vi "ULtravolt_Test_V1.3.vi"() -> ()   [LabVIEW 2022 SP3]
panel:
  out "UltraVolt Pout":dynamicdata(graph)=[{"t0"=timestamp(3793121458.353568 s since 1904-01-01), "dt"=0.004, "Y"=[0.002604330009442325, 0.0025504771878336083, 0.002568428128369847, 0.002532775426754479, 0.00251507366567535, 0.0024973719045962212, 0.0024973719045962212, 0.002550601777562163, 0.002568428128369847, 0.002586254479177531, 0.002604330009442325, 0.00275042932830334, 0.002604080829985215, 0.002358000431077182, 0.0020747622341868144, 0.001841629147424206, 0.0018114583938652624, 0.0017221920304739823, 0.0017667006224410674, 0.001737152817524899, 0.001737152817524899, 0.0016930179947434792, 0.0017518644251187055, 0.0017224412099310924, 0.0017224412099310924, 0.0016643423179271966, 0.0017667006224410674, 0.0017221920304739823, 0.0017667006224410674, 0.0017667006224410674, 0.0017221920304739823, 0.001856839113932233, 0.0019803876919247754, 0.002223114187786126, 0.0024607224851524124, 0.0027501801488462293, 0.00275042932830334, 0.0026222809499785644, 0.002676632130501502, 0.0026402318905148032, 0.0025504771878336083, 0.0026222809499785644, 0.002550601777562163, 0.002568428128369847, 0.002604330009442325, 0.002604330009442325, 0.002604330009442325, 0.002604330009442325, 0.002604330009442325, 0.002568178948912737, 0.002514949075946795, 0.002462217561895074, 0.0024796701435170925, 0.0024973719045962212, 0.002532775426754479, 0.0026404810699719133, 0.0026950814299519614, 0.0026950814299519614, 0.0025858807099918657, 0.0023233444472902545, 0.0020437193525279854, 0.001826419180916179, 0.0017964976068143457, 0.0017667006224410674, 0.0017964976068143457, 0.0017518644251187055, 0.0017812876403063187, 0.0017224412099310924, 0.0017077296023372858, 0.0016932671742005893, 0.001737152817524899, 0.0017224412099310924, 0.0017077296023372858, 0.0016930179947434792, 0.0017518644251187055, 0.0017518644251187055, 0.0018114583938652624, 0.001841629147424206, 0.0019333873053865884, 0.002172999058034062, 0.002392407235406999, 0.002658556600236708, 0.0028061509958403836, 0.0026952060196805167, 0.002658182831051042, 0.002658556600236708, 0.002604330009442325, 0.0025858807099918657, 0.002604330009442325, 0.0025863790689060863, 0.002586254479177531, 0.002604330009442325, 0.002586254479177531, 0.0026222809499785644, 0.002568178948912737, 0.002568428128369847, 0.002568178948912737, 0.00251507366567535, 0.0024796701435170925, 0.002514949075946795], "attributes"=variant("NI_ChannelName"=variant(string "Eout (Ultravolt)"), "NI_UnitDescription"=variant(string "E-Volts"))}]
  out "UltraVolt Eout":dynamicdata(graph)=[{"t0"=timestamp(3793121458.353568 s since 1904-01-01), "dt"=0.004, "Y"=[-4.674759833142161, -4.642537981271744, -4.642537981271744, -4.578094277530909, -4.578094277530909, -4.545872425660491, -4.578094277530909, -4.610316129401326, -4.610316129401326, -4.610316129401326, -4.642537981271744, -4.771425388753414, -4.706981685012579, -4.481428721919656, -4.255875758826733, -3.9336572401225567, -3.901435388252139, -3.836991684511304, -3.836991684511304, -3.8047698326408863, -3.8047698326408863, -3.8047698326408863, -3.8047698326408863, -3.7725479807704687, -3.8047698326408863, -3.740326128900051, -3.836991684511304, -3.836991684511304, -3.836991684511304, -3.836991684511304, -3.740326128900051, -3.9336572401225567, -4.0303227957338095, -4.28809761069715, -4.416985018178821, -4.739203536882997, -4.803647240623832, -4.642537981271744, -4.771425388753414, -4.739203536882997, -4.642537981271744, -4.642537981271744, -4.610316129401326, -4.610316129401326, -4.642537981271744, -4.674759833142161, -4.674759833142161, -4.674759833142161, -4.674759833142161, -4.674759833142161, -4.545872425660491, -4.545872425660491, -4.513650573790073, -4.545872425660491, -4.578094277530909, -4.674759833142161, -4.706981685012579, -4.771425388753414, -4.706981685012579, -4.481428721919656, -4.15921020321548, -3.9336572401225567, -3.8692135363817215, -3.836991684511304, -3.8692135363817215, -3.8047698326408863, -3.8047698326408863, -3.8047698326408863, -3.8047698326408863, -3.7725479807704687, -3.8047698326408863, -3.8047698326408863, -3.740326128900051, -3.8047698326408863, -3.8047698326408863, -3.836991684511304, -3.901435388252139, -3.9336572401225567, -3.9658790919929743, -4.1914320550858974, -4.416985018178821, -4.674759833142161, -4.868090944364667, -4.739203536882997, -4.642537981271744, -4.739203536882997, -4.642537981271744, -4.578094277530909, -4.674759833142161, -4.642537981271744, -4.674759833142161, -4.674759833142161, -4.674759833142161, -4.642537981271744, -4.674759833142161, -4.642537981271744, -4.674759833142161, -4.578094277530909, -4.513650573790073, -4.545872425660491], "attributes"=variant("NI_ChannelName"=variant(string "Eout (Ultravolt)"), "NI_UnitDescription"=variant(string "E-Volts"))}]
  out "UltraVolt Iout":dynamicdata(graph)=[{"t0"=timestamp(3793121458.355568 s since 1904-01-01), "dt"=0.004, "Y"=[-0.5571045577526093, -0.549371313303709, -0.5532379355281591, -0.5532379355281591, -0.549371313303709, -0.549371313303709, -0.5455046910792589, -0.5532379355281591, -0.5571045577526093, -0.5609711799770594, -0.5609711799770594, -0.5764376688748598, -0.5532379355281591, -0.5261715799570084, -0.48750535771250725, -0.4681722465902567, -0.4643056243658066, -0.44883913546800613, -0.46043900214135647, -0.45657237991690636, -0.45657237991690636, -0.444972513243556, -0.46043900214135647, -0.45657237991690636, -0.45270575769245625, -0.444972513243556, -0.46043900214135647, -0.44883913546800613, -0.46043900214135647, -0.46043900214135647, -0.46043900214135647, -0.4720388688147068, -0.49137197993695736, -0.5184383355081081, -0.5571045577526093, -0.5803042910993099, -0.5725710466504097, -0.5648378022015095, -0.5609711799770594, -0.5571045577526093, -0.549371313303709, -0.5648378022015095, -0.5532379355281591, -0.5571045577526093, -0.5609711799770594, -0.5571045577526093, -0.5571045577526093, -0.5571045577526093, -0.5571045577526093, -0.549371313303709, -0.5532379355281591, -0.5416380688548088, -0.549371313303709, -0.549371313303709, -0.5532379355281591, -0.5648378022015095, -0.5725710466504097, -0.5648378022015095, -0.549371313303709, -0.5184383355081081, -0.49137197993695736, -0.4643056243658066, -0.4643056243658066, -0.46043900214135647, -0.4643056243658066, -0.46043900214135647, -0.4681722465902567, -0.45270575769245625, -0.44883913546800613, -0.44883913546800613, -0.45657237991690636, -0.45270575769245625, -0.45657237991690636, -0.444972513243556, -0.46043900214135647, -0.45657237991690636, -0.4643056243658066, -0.4681722465902567, -0.48750535771250725, -0.5184383355081081, -0.5416380688548088, -0.5687044244259596, -0.5764376688748598, -0.5687044244259596, -0.5725710466504097, -0.5609711799770594, -0.5609711799770594, -0.5648378022015095, -0.5571045577526093, -0.5571045577526093, -0.5532379355281591, -0.5571045577526093, -0.5532379355281591, -0.5648378022015095, -0.549371313303709, -0.5532379355281591, -0.549371313303709, -0.549371313303709, -0.549371313303709, -0.5532379355281591], "attributes"=variant("NI_ChannelName"=variant(string "Iout (Ultravolt)"), "NI_UnitDescription"=variant(string "mAmps"))}]
  out "Spark?":bool
  in  "Auto Spark":T1={"Start Time, sec"=1.0, "EndTime, sec"=3.0}
  out "Current Frame\n(Auto)":i32=10
  in  "Auto Frame \nWait\nState (ms)":i32=2
  in  "Maximum Run \nTime, Sec (Auto)":dbl=4.0
  in  "Manual Abort":bool
  out "Current Run time,\nsec (Auto)":dbl=4.020400000001246
  in  "Auto Firing\nCount Down Time\n(SECONDS)":dbl=5.0
  out "Auto Firing\nCount Down":i32 format="%#.1f"
  in  "Maximum Run \nTime, Sec \n(Manual)":dbl=15.0
  out "Current Frame":i32=38
  in  "Manual Frame Wait\nState (ms)":i32=2
  in  "Test Spark Path":bool
  out "Current Run time,\nsec (Manual)":dbl=15.238100000002305
  in  "stop":bool
  in  "error in (no error)":errorcluster
  out "AutoRun\nIndicator":bool
  in  "Control Action":bool
  in  "Log File Frames \nFor Each  Read":i32=100
  in  "Log File Read \nSample Rate, SPS":dbl=250.0
  out "Epoch Total Seconds \nfrom Midnight\n(Beginning of Run)":dbl=53443.1215 format="%.4f"
  in  "Ultravolt Output Folder Path":path=path "C:/Users/nasa PC/Desktop/Estes/test_data"
  out "UltraVolt Log File Path":path=path "C:/Users/nasa PC/Desktop/Estes/test_data/test_MyDAQ_Ultravolt_3_12_2024_2.50 PM.lvm"
  in  "Ultravolt Output File Name":string="test_MyDAQ_Ultravolt"
  in  "Ultravolt Output\nFile Appendage":string=".lvm"
  in  "Start VI":bool
  out "Waiting \nfor Start":bool=TRUE
  # "Auto Sequence"
  # "Manual Sequence Control"
  # "Manual"
  # "Auto"
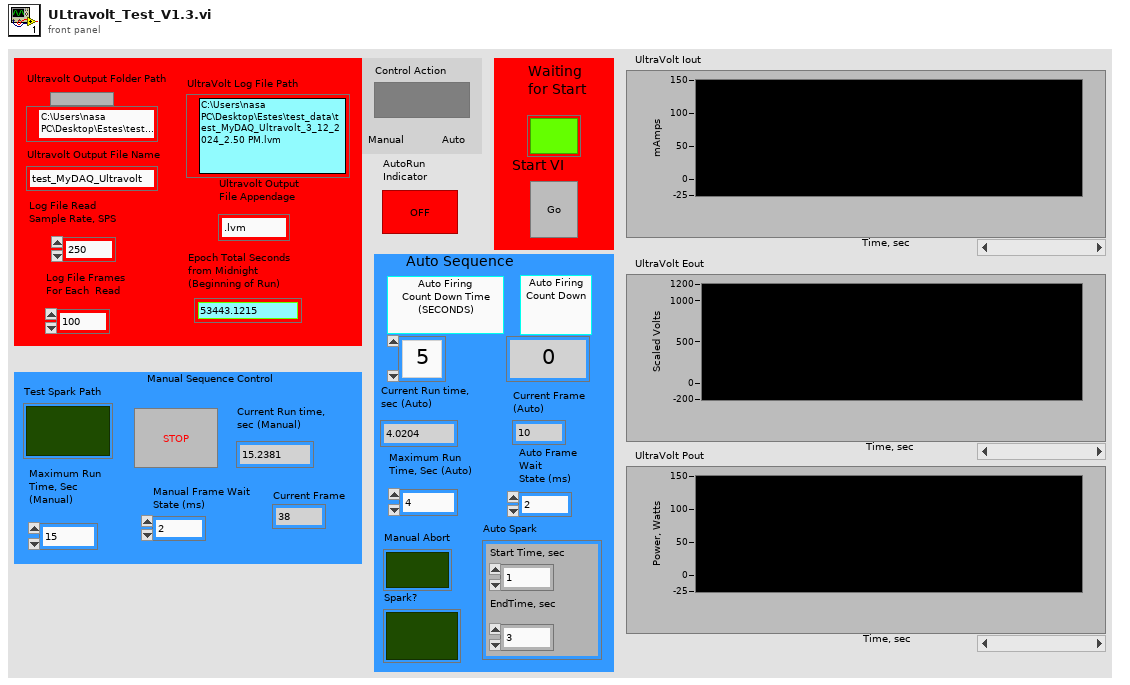
[diagram p1: front panel]
types:
  T1 = cluster{"Start Time, sec":dbl, "EndTime, sec":dbl}
  T2 = cluster{"Modulus":dbl, "Number of\nComplete Cycles":dbl}
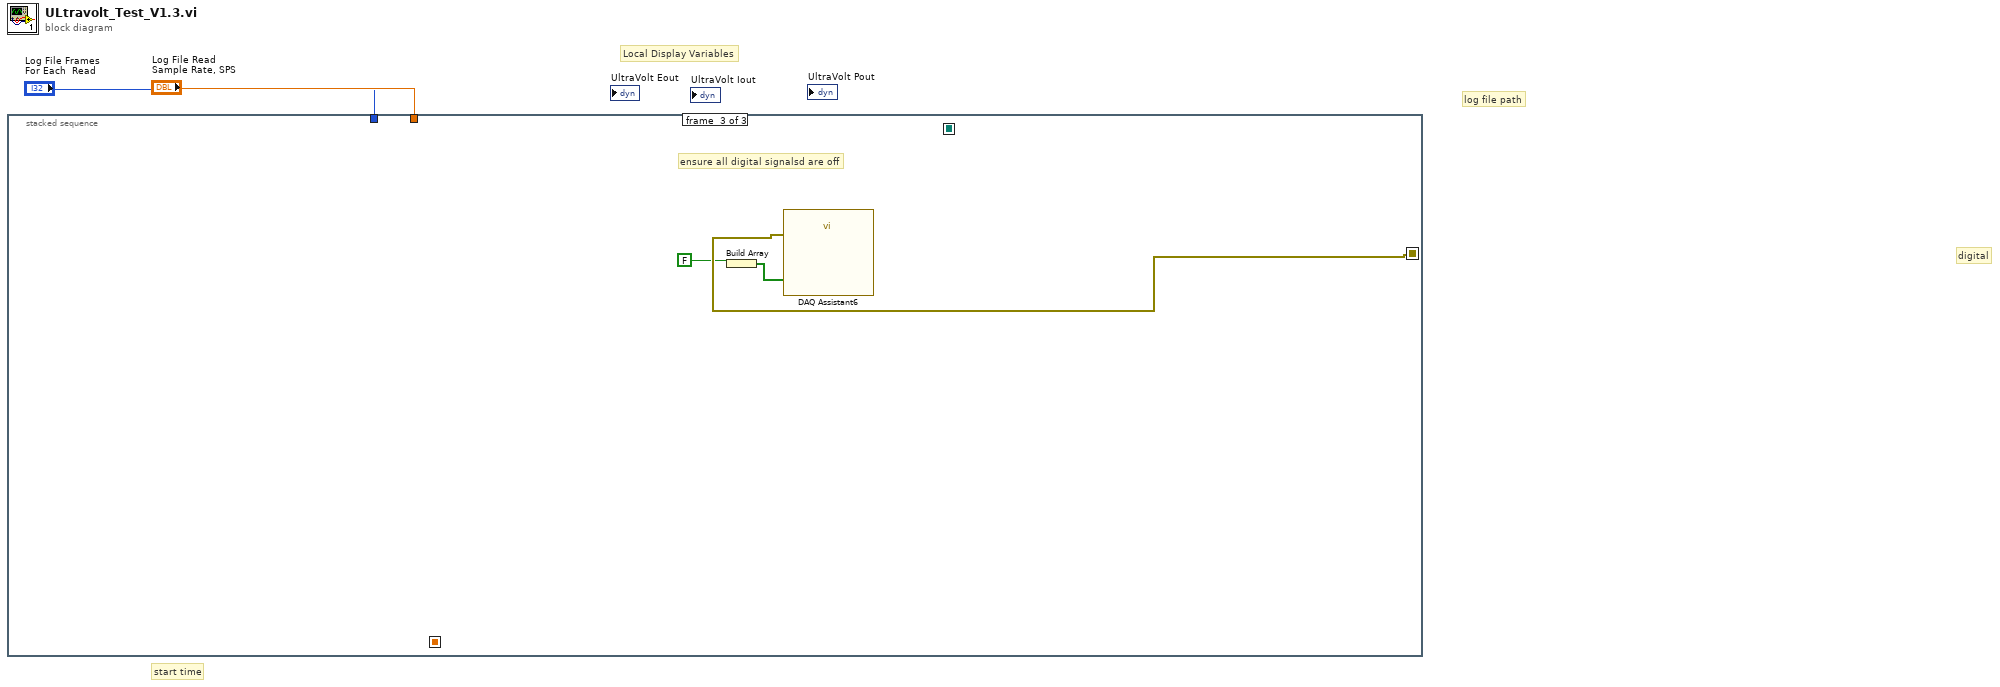
[diagram p0: block diagram]
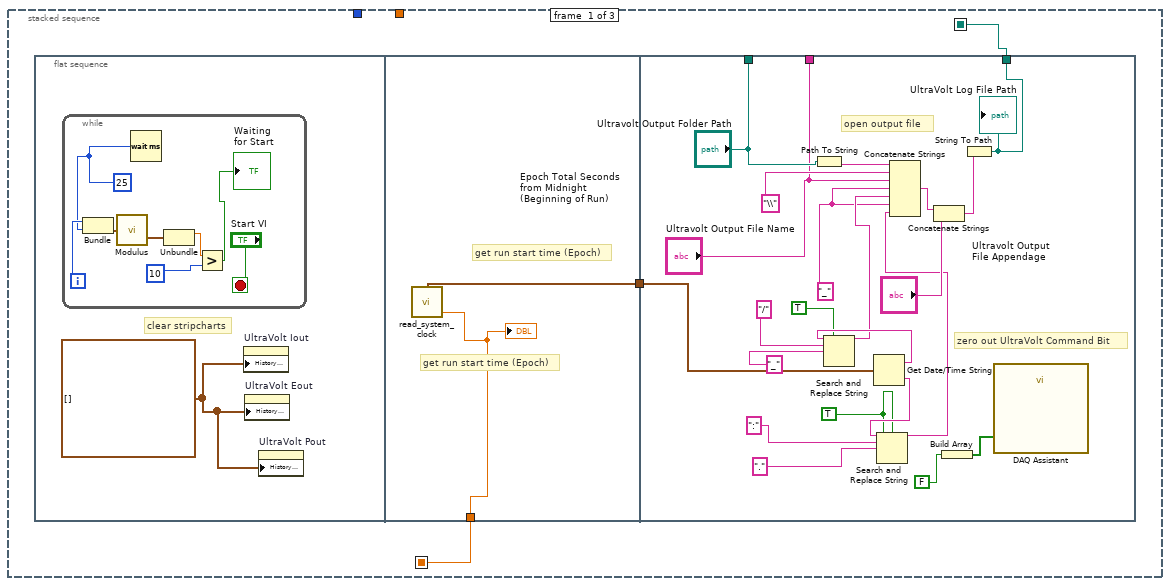
[diagram p2: hidden frame]
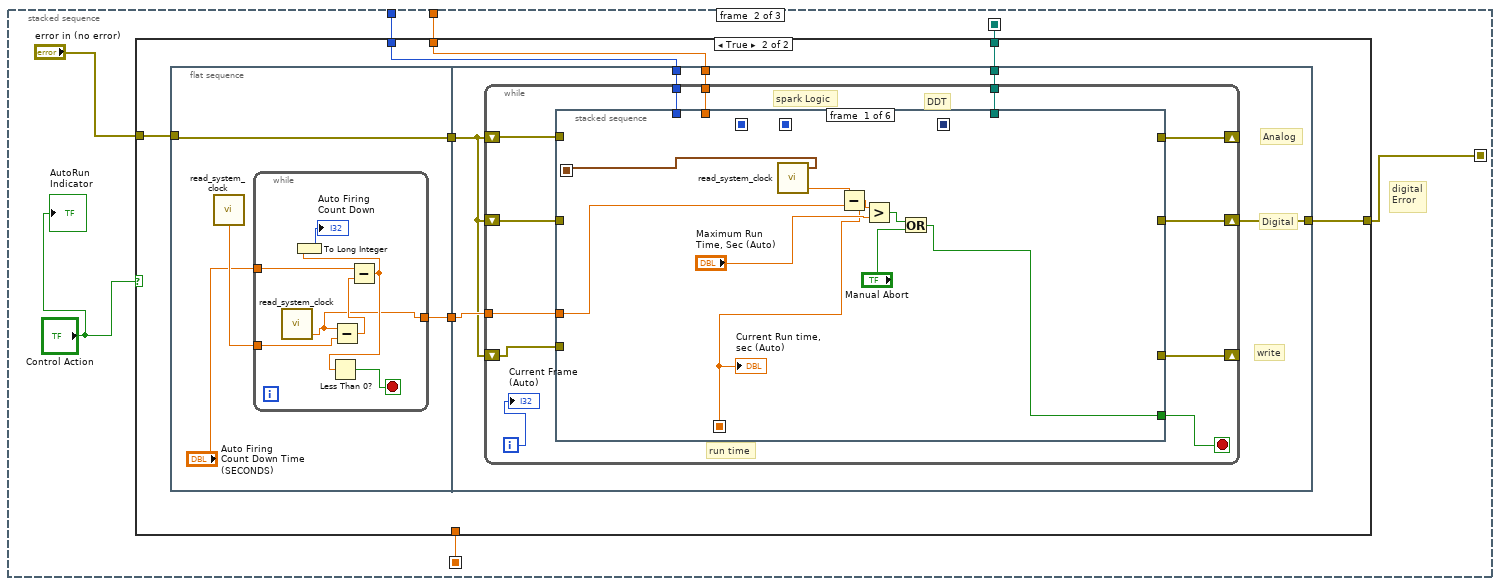
[diagram p3: hidden frame]
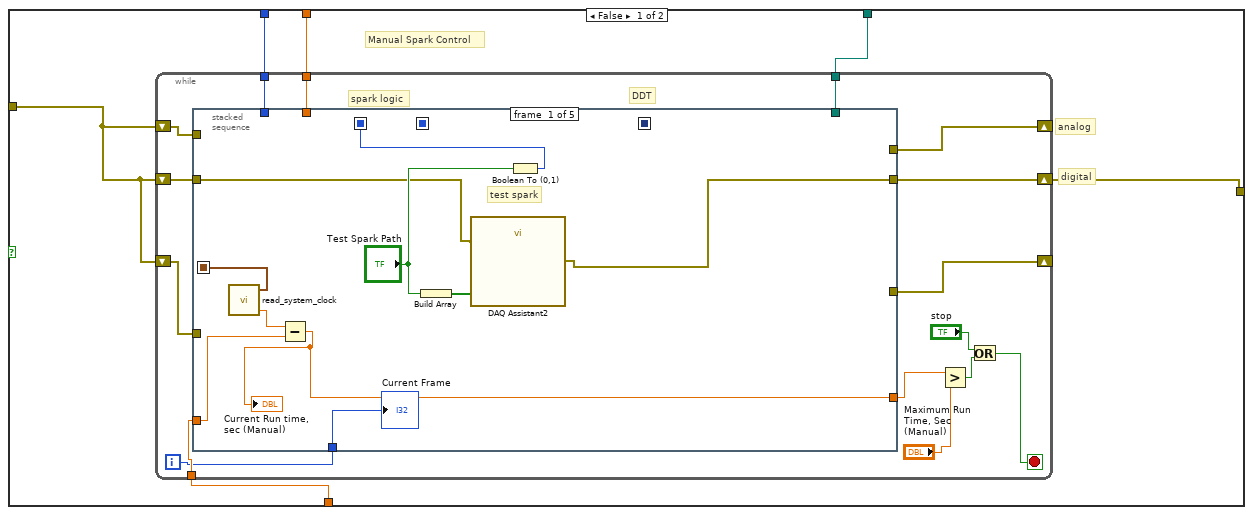
[diagram p4: hidden frame]
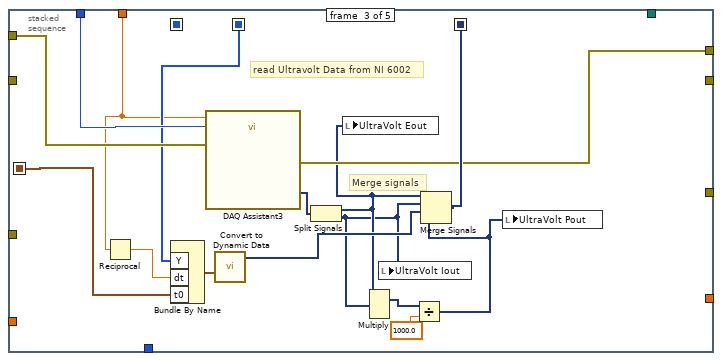
[diagram p6: hidden frame]
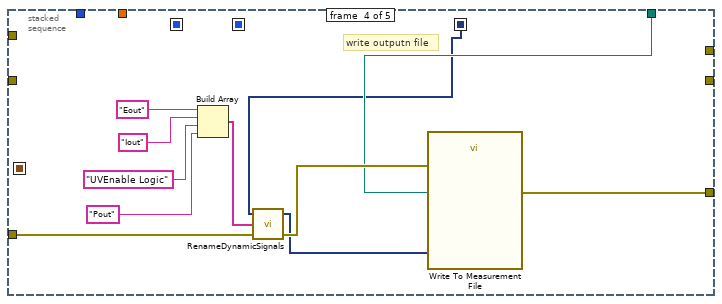
[diagram p7: hidden frame]
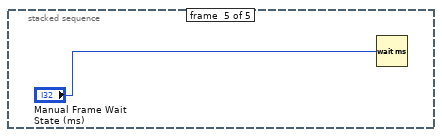
[diagram p8: hidden frame]
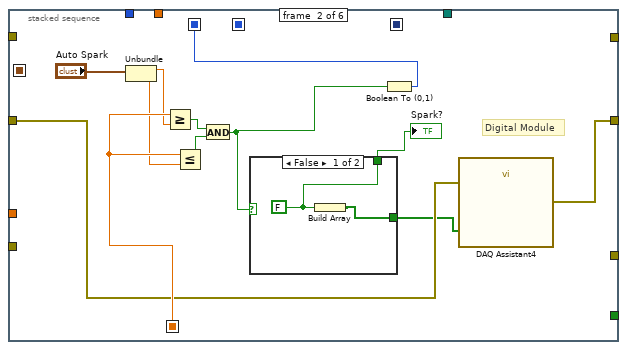
[diagram p9: hidden frame]
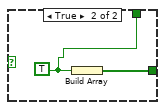
[diagram p10: hidden frame]
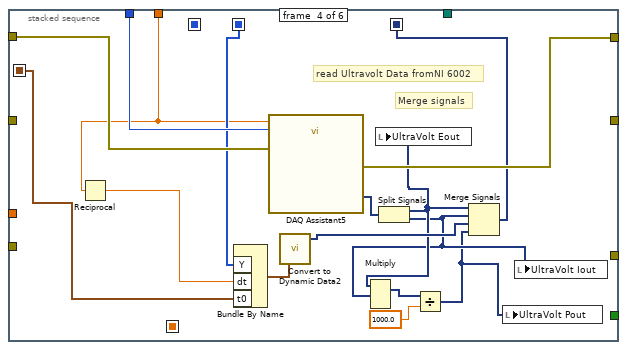
[diagram p12: hidden frame]
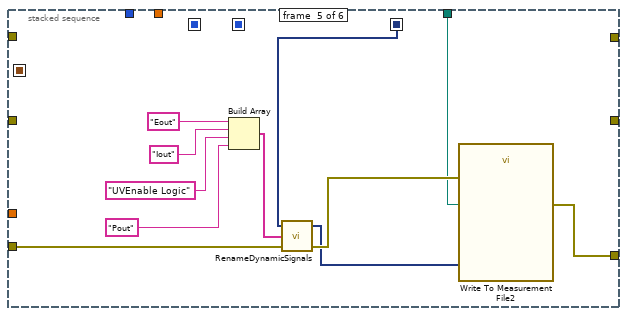
[diagram p13: hidden frame]
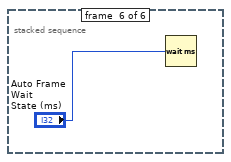
[diagram p14: hidden frame]
diagram:
  # "Local Display Variables"
  # "digital"
  # "log file path"
  # "start time"
  n1 = stacked-sequence {
    seq-local: [w4 _ _] -> [_ w40 _]
    seq-local: [w3 _ _] -> [_ w44 _]
    seq-local: [_ w39 _] -> [_ _ w204]
    tunnel: "Log File Read \nSample Rate, SPS" -> [_ w42 _]
    tunnel: "Log File Frames \nFor Each  Read" -> [_ w41 _]
    frame #0 {
      n2 = flat-sequence {
        tunnel: [w16] -> w5
        tunnel: [w15] -> w3
        tunnel: [w25] -> w4
        tunnel: w5 -> [w26]
        tunnel: ["Ultravolt Output Folder Path"] -> _
        tunnel: ["Ultravolt Output File Name"] -> _
        frame #0 {
          w6 = waveform(dbl)[] []
          # "clear stripcharts"
          n3 = while {
            i -> [w13]
            stop <- "Start VI" stop-if-true
            w8 = u32 25
            n4 = Bundle(w13, w8) -> (w9:cluster{i32, u32})  [unwired: 1 in]
            n5 = call "Modulus.vi"("Input"=w9) -> ("Output"=w12:T2)
            n6 = Wait (ms)(milliseconds to wait=w8) -> ()  [unwired: 1 out]
            n7 = Unbundle(w12) -> ("Modulus"=w11:dbl)  [unwired: 1 out]
            n8 = Greater?(x=w11, y=10) -> (0:→"Waiting \nfor Start":bool)
          }
          n9 = property on="UltraVolt Iout" class="WFChart (strict)"("History Data"=w6) -> ()  [unwired: 2 in, 2 out]
          n10 = property on="UltraVolt Eout" class="WFChart (strict)"("History Data"=w6) -> ()  [unwired: 2 in, 2 out]
          n11 = property on="UltraVolt Pout" class="WFChart (strict)"("History Data"=w6) -> ()  [unwired: 2 in, 2 out]
        }
        frame #1 {
          # "get run start time (Epoch)"
          # "get run start time (Epoch)"
          n12 = call "read_system_clock.vi"() -> ("Total Seconds from Midnight"=w15:dbl, "LABVIEW TIME STAMP"=w16:timestamp)  [unwired: 1 out]
          "Epoch Total Seconds \nfrom Midnight\n(Beginning of Run)" <- w15
        }
        frame #2 {
          w27 = TRUE
          w31 = "_"
          # "zero out UltraVolt Command Bit"
          # "open output file"
          n13 = Path To String(path="Ultravolt Output Folder Path") -> (string=w37:string)
          n14 = Get Date/Time String(seconds (now)=w26) -> (date string=w36:string, time string=w30:string)  [unwired: 2 in]
          n15 = Search and Replace String(replace all?=TRUE, input string=w36, search string="/", replace string="_") -> (result string=w32:string)  [unwired: 4 in, 3 out]
          n16 = Search and Replace String(replace all?=w27, case sensitive?=w27, input string=w30, search string=":", replace string=".") -> (result string=w17:string)  [unwired: 3 in, 3 out]
          n17 = Concatenate Strings(w37, "\\", "Ultravolt Output File Name", w31, w32, w31, w17) -> (w21:string)
          n18 = Concatenate Strings(w21, "Ultravolt Output\nFile Appendage") -> (w24:string)
          n19 = Build Array(FALSE) -> (w18:bool[])
          n20 = String To Path(string=w24) -> (path=w25:path)
          "UltraVolt Log File Path" <- w25
          n21 = call "DAQ Assistant"("data"=w18) -> ()  [unwired: 17 in, 2 out]
        }
      }
    }
    frame #1 {
      # "digital\nError"
      n22 = case shown="True" "Control Action" {
        tunnel: w44 -> [w51 _]
        tunnel: "error in (no error)" -> [w47 w114]
        tunnel: w42 -> [w50 w112]
        tunnel: w41 -> [w49 w113]
        tunnel: w40 -> [w48 w111]
        tunnel: [w46 w110] -> w39
        frame False {
          # "digital"
          # "analog"
          # "Manual Spark Control"
          n23 = while {
            tunnel: w51 -> [w67]
            shift-right: [w52] -> _
            shift-left: w47 -> [w62]
            shift-right: [w60] -> w46
            shift-left: w47 -> [w61]
            tunnel: w50 -> [w59]
            tunnel: w49 -> [w58]
            tunnel: w48 -> [w57]
            shift-right: [w53] -> _
            shift-left: w47 -> [w54]
            i -> [w56]
            stop <- w63 stop-if-true
            # "DDT"
            # "spark logic"
            n24 = stacked-sequence {
              seq-local: [w72 _ _ _ _] -> [_ w79 _ _ _]
              seq-local: [w69 _ _ _ _] -> [_ _ w93 _ _]
              seq-local: [_ _ w92 _ _] -> [_ _ _ w103 _]
              seq-local: [_ w78 _ _ _] -> [_ _ w91 _ _]
              tunnel: w67 -> [w76 _ _ _ _]
              tunnel: [w75 _ _ _ _] -> w66
              tunnel: w62 -> [_ _ w97 _ _]
              tunnel: w61 -> [w71 _ _ _ _]
              tunnel: [w70 _ _ _ _] -> w60
              tunnel: w59 -> [_ _ w89 _ _]
              tunnel: w58 -> [_ w80 w96 _ _]
              tunnel: w57 -> [_ _ _ w106 _]
              tunnel: [_ _ _ w101 _] -> w53
              tunnel: w56 -> [w68 _ _ _ _]
              tunnel: w54 -> [_ _ _ w100 _]
              tunnel: [_ _ w90 _ _] -> w52
              frame #0 {
                # "test spark"
                n25 = call "read_system_clock.vi"() -> ("Total Seconds from Midnight"=w77:dbl, "LABVIEW TIME STAMP"=w69:timestamp)  [unwired: 1 out]
                n26 = Subtract(x=w77, y=w76) -> (x-y=w75:dbl)
                "Current Run time,\nsec (Manual)" <- w75
                n27 = Build Array("Test Spark Path") -> (w74:bool[])
                n28 = call "DAQ Assistant2"("data"=w74, "error in"=w71) -> ("error out"=w70:errorcluster)  [unwired: 16 in, 1 out]
                n29 = Boolean To (0,1)(Boolean="Test Spark Path") -> (0, 1=w72:i16)
                "Current Frame" <- w68
              }
              frame #1 {
                n30 = for {
                  N: w80 -> [_]
                  tunnel: w79 -> [w81]
                  tunnel: [w81] -> w78 mode=indexing
                  # "fill out logic buffer"
                }
              }
              frame #2 {
                # "Merge signals"
                # "read Ultravolt Data from NI 6002"
                n31 = Reciprocal(x=w89) -> (1/x=w88:dbl)
                n32 = Bundle By Name("Y"=w91, "dt"=w88, "t0"=w93) -> (w94:waveform(i16))  [unwired: 1 in]
                n33 = call "DAQ Assistant3"("rate"=w89, "number of samples"=w96, "error in"=w97) -> ("data"=w95:dynamicdata, "error out"=w90:errorcluster)  [unwired: 13 in, 2 out]
                n34 = call "Convert to Dynamic Data"("Waveform"=w94) -> ("Dynamic Data Type"=w87:dynamicdata)  [unwired: 3 in]
                n35 = Split Signals(w95) -> (w86:dynamicdata, w85:dynamicdata)  [unwired: 2 in]
                n36 = local write "UltraVolt Eout"(w86) -> ()
                n37 = Multiply(1:w85, 2:w86) -> (0:w84:dynamicdata)  [unwired: 1 in, 1 out]
                n38 = local write "UltraVolt Iout"(w85) -> ()
                n39 = Divide(x=w84, y=1000.0) -> (x/y=w82:dynamicdata)
                n40 = Merge Signals(w86, w85, w87, w82) -> (w92:dynamicdata)
                n41 = local write "UltraVolt Pout"(w82) -> ()
              }
              frame #3 {
                # "write outputn file"
                n42 = Build Array("Eout", "Iout", "UVEnable Logic", "Pout") -> (w102:string[])
                n43 = call "RenameDynamicSignals.vi"("error in"=w100, "New Signal Names"=w102, "Dynamic Data In"=w103) -> ("error out"=w108:errorcluster, "Dynamic Data Out"=w107:dynamicdata)  [unwired: 1 in]
                n44 = call "Write To Measurement File"("Signals"=w107, "error in (no error)"=w108, "Filename"=w106) -> ("error out"=w101:errorcluster)  [unwired: 14 in, 2 out]
              }
              frame #4 {
                n45 = Wait (ms)(milliseconds to wait="Manual Frame Wait\nState (ms)") -> ()  [unwired: 1 out]
              }
            }
            n46 = Greater?(x=w66, y="Maximum Run \nTime, Sec \n(Manual)") -> (0:w64:bool)
            n47 = Or(x="stop", y=w64) -> (x .or. y?=w63:bool)
          }
        }
        frame True {
          n48 = flat-sequence {
            tunnel: [w118] -> w116
            tunnel: [w117] -> w115
            tunnel: w114 -> [w117]
            tunnel: w116 -> [w133]
            tunnel: w115 -> [w130]
            tunnel: w113 -> [w132]
            tunnel: w112 -> [w131]
            tunnel: w111 -> [w129]
            tunnel: [w128] -> w110
            frame #0 {
              n49 = call "read_system_clock.vi"() -> ("Total Seconds from Midnight"=w120:dbl)  [unwired: 2 out]
              n50 = while {
                tunnel: w120 -> [w127]
                tunnel: "Auto Firing\nCount Down Time\n(SECONDS)" -> [w126]
                tunnel: [w121] -> w118
                stop <- w124 stop-if-true
                n51 = call "read_system_clock.vi"() -> ("Total Seconds from Midnight"=w121:dbl)  [unwired: 2 out]
                n52 = Subtract(x=w121, y=w127) -> (x-y=w123:dbl)
                n53 = Subtract(x=w126, y=w123) -> (x-y=w125:dbl)
                n54 = To Long Integer(number=w125) -> (32bit integer=→"Auto Firing\nCount Down":i32)
                n55 = Less Than 0?(x=w125) -> (x < 0?=w124:bool)
              }
            }
            frame #1 {
              # "write"
              # "Analog"
              # "Digital"
              n56 = while {
                shift-right: [w143] -> _
                shift-left: w130 -> [w142]
                tunnel: w133 -> [w145]
                shift-right: [w139] -> w128
                shift-left: w130 -> [w140]
                tunnel: w132 -> [w138]
                tunnel: w131 -> [w137]
                shift-right: [w134] -> _
                shift-left: w130 -> [w136]
                tunnel: w129 -> [w135]
                i -> [w141]
                stop <- w144 stop-if-true
                # "DDT"
                # "spark Logic"
                # "run time"
                n57 = stacked-sequence {
                  seq-local: [w147 _ _ _ _ _] -> [_ w164 _ _ _ _]
                  seq-local: [_ w157 _ _ _ _] -> [_ _ w172 _ _ _]
                  seq-local: [_ _ w171 _ _ _] -> [_ _ _ w185 _ _]
                  seq-local: [_ _ _ w183 _ _] -> [_ _ _ _ w194 _]
                  seq-local: [w146 _ _ _ _ _] -> [_ _ _ w180 _ _]
                  tunnel: w145 -> [w150 _ _ _ _ _]
                  tunnel: [w148 _ _ _ _ _] -> w144
                  tunnel: [_ _ _ w184 _ _] -> w143
                  tunnel: w142 -> [_ _ _ w187 _ _]
                  tunnel: w140 -> [_ w160 _ _ _ _]
                  tunnel: [_ w159 _ _ _ _] -> w139
                  tunnel: w138 -> [_ _ w170 w186 _ _]
                  tunnel: w137 -> [_ _ _ w182 _ _]
                  tunnel: w136 -> [_ _ _ _ w195 _]
                  tunnel: w135 -> [_ _ _ _ w193 _]
                  tunnel: [_ _ _ _ w192 _] -> w134
                  frame #0 {
                    n58 = call "read_system_clock.vi"() -> ("Total Seconds from Midnight"=w151:dbl, "LABVIEW TIME STAMP"=w146:timestamp)  [unwired: 1 out]
                    n59 = Subtract(x=w151, y=w150) -> (x-y=w147:dbl)
                    "Current Run time,\nsec (Auto)" <- w147
                    n60 = Greater?(x=w147, y="Maximum Run \nTime, Sec (Auto)") -> (0:w152:bool)
                    n61 = Or(x=w152, y="Manual Abort") -> (x .or. y?=w148:bool)
                  }
                  frame #1 {
                    # "Digital Module"
                    n62 = Unbundle("Auto Spark") -> ("Start Time, sec"=w163:dbl, "EndTime, sec"=w156:dbl)
                    n63 = Greater Or Equal?(x=w164, y=w163) -> (x >= y?=w162:bool)
                    n64 = Less Or Equal?(x=w164, y=w156) -> (x <= y?=w161:bool)
                    n65 = And(x=w162, y=w161) -> (x .and. y?=w158:bool)
                    n66 = case shown="False" w158 {
                      tunnel: [w167 w169] -> w155
                      tunnel: [w166 w168] -> w154
                      frame False {
                        w166 = FALSE
                        n67 = Build Array(w166) -> (w167:bool[])
                      }
                      frame True {
                        w168 = TRUE
                        n68 = Build Array(w168) -> (w169:bool[])
                      }
                    }
                    "Spark?" <- w154
                    n69 = Boolean To (0,1)(Boolean=w158) -> (0, 1=w157:i16)
                    n70 = call "DAQ Assistant4"("data"=w155, "error in"=w160) -> ("error out"=w159:errorcluster)  [unwired: 16 in, 1 out]
                  }
                  frame #2 {
                    n71 = for {
                      N: w170 -> [_]
                      tunnel: w172 -> [w173]
                      tunnel: [w173] -> w171 mode=indexing
                      # "fill out logic buffer"
                    }
                  }
                  frame #3 {
                    # "Merge signals"
                    # "read Ultravolt Data fromNI 6002"
                    n72 = Reciprocal(x=w182) -> (1/x=w181:dbl)
                    n73 = Bundle By Name("Y"=w185, "dt"=w181, "t0"=w180) -> (w188:waveform(i16))  [unwired: 1 in]
                    n74 = call "DAQ Assistant5"("rate"=w182, "number of samples"=w186, "error in"=w187) -> ("data"=w189:dynamicdata, "error out"=w184:errorcluster)  [unwired: 13 in, 2 out]
                    n75 = call "Convert to Dynamic Data2"("Waveform"=w188) -> ("Dynamic Data Type"=w179:dynamicdata)  [unwired: 3 in]
                    n76 = Split Signals(w189) -> (w176:dynamicdata, w175:dynamicdata)  [unwired: 2 in]
                    n77 = Multiply(1:w175, 2:w176) -> (0:w178:dynamicdata)  [unwired: 1 in, 1 out]
                    n78 = local write "UltraVolt Eout"(w176) -> ()
                    n79 = Divide(x=w178, y=1000.0) -> (x/y=w174:dynamicdata)
                    n80 = Merge Signals(w176, w175, w179, w174) -> (w183:dynamicdata)
                    n81 = local write "UltraVolt Pout"(w174) -> ()
                    n82 = local write "UltraVolt Iout"(w175) -> ()
                  }
                  frame #4 {
                    n83 = Build Array("Eout", "Iout", "UVEnable Logic", "Pout") -> (w196:string[])
                    n84 = call "RenameDynamicSignals.vi"("error in"=w195, "New Signal Names"=w196, "Dynamic Data In"=w194) -> ("error out"=w200:errorcluster, "Dynamic Data Out"=w199:dynamicdata)  [unwired: 1 in]
                    n85 = call "Write To Measurement File2"("Signals"=w199, "error in (no error)"=w200, "Filename"=w193) -> ("error out"=w192:errorcluster)  [unwired: 14 in, 2 out]
                  }
                  frame #5 {
                    n86 = Wait (ms)(milliseconds to wait="Auto Frame \nWait\nState (ms)") -> ()  [unwired: 1 out]
                  }
                }
                "Current Frame\n(Auto)" <- w141
              }
            }
          }
        }
      }
      "AutoRun\nIndicator" <- "Control Action"
    }
    frame #2 {
      # "ensure all digital signalsd are off"
      n87 = Build Array(FALSE) -> (w202:bool[])
      n88 = call "DAQ Assistant6"("data"=w202, "error in"=w204) -> ()  [unwired: 16 in, 2 out]
    }
  }
